vi "Calculate no of Hist bins.vi"(0 "Mean":dbl, 1 "Standard Deviation":dbl, 2 "Time Trace":dbl[](array[numeric]), 3 "Shift Input":T1, 4 "Number of Bins per Sigma":dbl=50.0 format="%#_13g") -> (6 "Shift Output":T1)   [LabVIEW 2022 SP3]
uses:
  Controls/Shift_Cluster.ctl
  Globals/Meas_global.vi
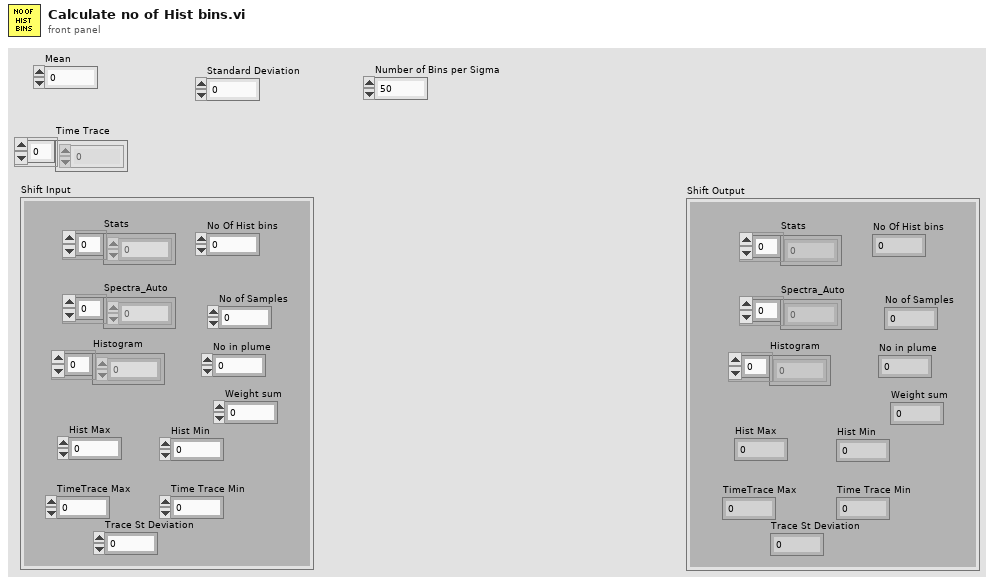
[diagram p1: front panel]
types:
  T1 = typedef "Shift_Cluster.ctl" = cluster{"Stats":dbl[], "Spectra_Auto":dbl[], "Histogram":dbl[], "Hist Max":dbl, "Hist Min":dbl, "No of Samples":i32, "No in plume":i32, "Weight sum":dbl, "No Of Hist bins":i32, "TimeTrace Max":dbl, "Time Trace Min":dbl, "Trace St Deviation":dbl}
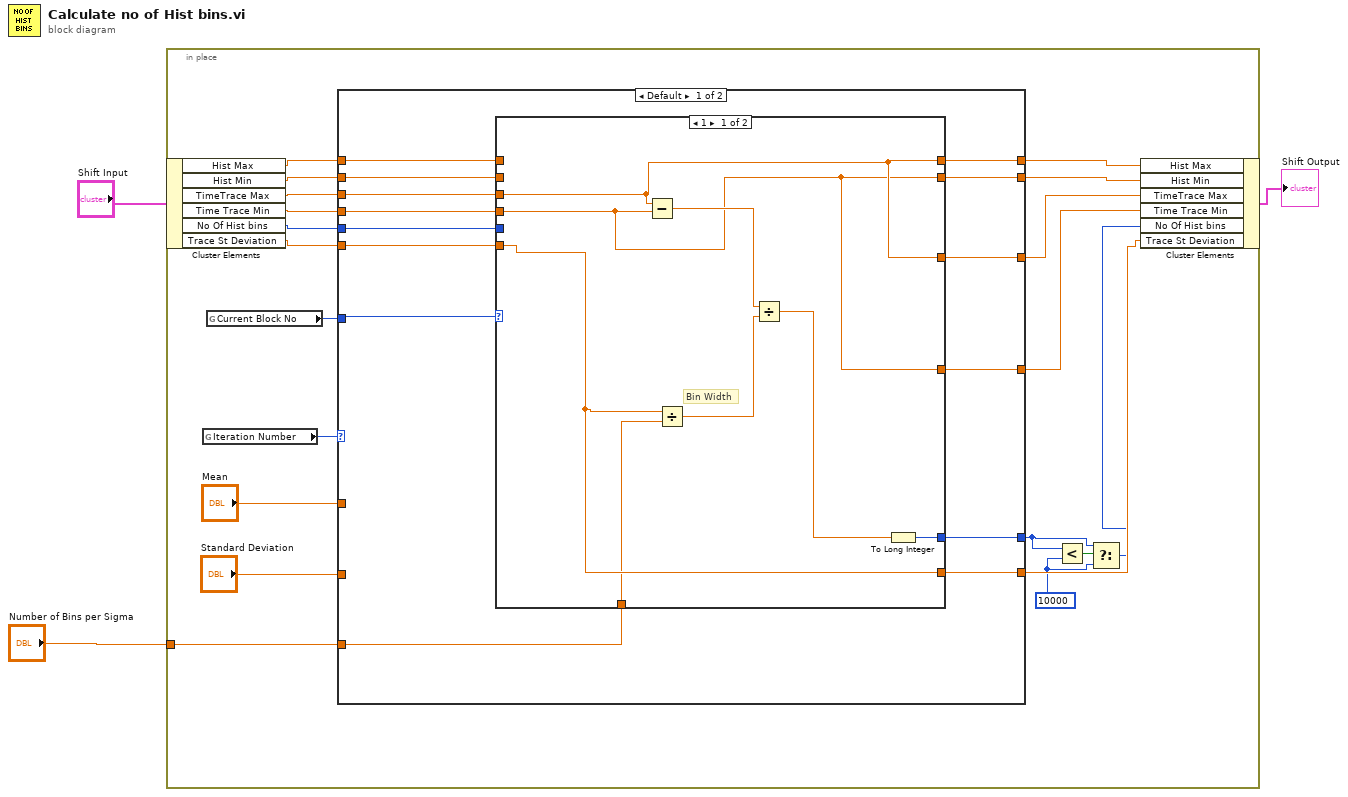
[diagram p0: block diagram]
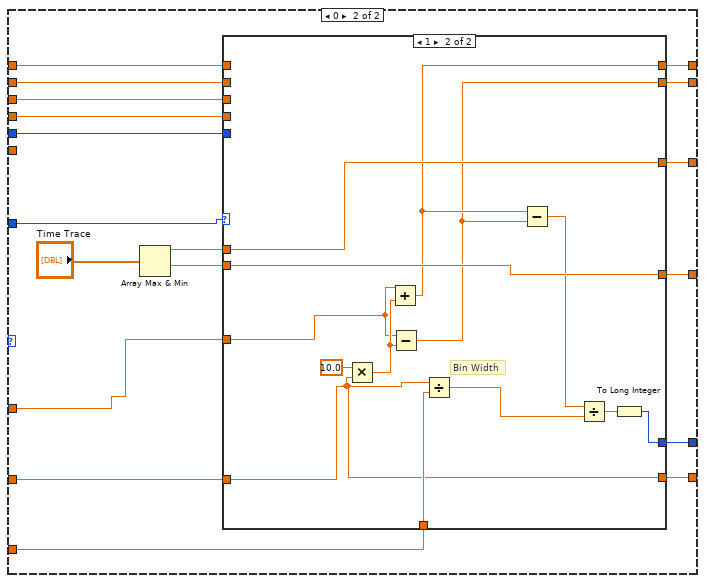
[diagram p3: hidden frame]
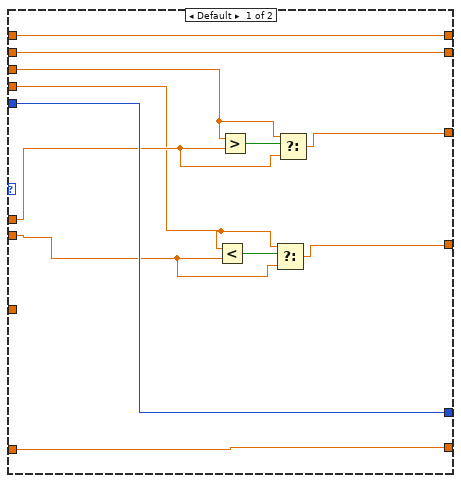
[diagram p4: hidden frame]
diagram:
  n1 = in-place {
    in-place-border: "Number of Bins per Sigma" -> [w10]
    w5 = 10000 ("y")
    n2 = in-place-cluster #1("Shift Input") -> ("Hist Max"=w17:dbl, "Hist Min"=w16:dbl, "TimeTrace Max"=w14:dbl, "Time Trace Min"=w13:dbl, "No Of Hist bins"=w15:i32, "Trace St Deviation"=w11:dbl)
    n3 = global read "Meas_global.vi" "Iteration Number"() -> (w23:i32)
    n4 = global read "Meas_global.vi" "Current Block No"() -> (w22:i32)
    n5 = case shown="Default" w23 {
      tunnel: w22 -> [w37 w68]
      tunnel: [w29 w67] -> w19
      tunnel: [w32 w66] -> w18
      tunnel: [w33 w63] -> w6
      tunnel: [w28 w62] -> w21
      tunnel: [w25 w61] -> w20
      tunnel: w17 -> [w27 w60]
      tunnel: w16 -> [w26 w59]
      tunnel: w15 -> [w34 w58]
      tunnel: w14 -> [w30 w57]
      tunnel: w13 -> [w31 w56]
      tunnel: [w36 w55] -> w12
      tunnel: w11 -> [w35 _]
      tunnel: w10 -> [w24 w54]
      tunnel: "Mean" -> [_ w53]
      tunnel: "Standard Deviation" -> [_ w52]
      frame Default {
        n6 = case shown="1" w37 {
          tunnel: [w41 w51] -> w36
          tunnel: w35 -> [w41 w51]
          tunnel: w34 -> [_ w50]
          tunnel: [w42 w50] -> w33
          tunnel: [w39 w49] -> w32
          tunnel: w31 -> [w39 w49]
          tunnel: w30 -> [w40 w48]
          tunnel: [w40 w48] -> w29
          tunnel: [w40 w47] -> w28
          tunnel: w27 -> [_ w47]
          tunnel: w26 -> [_ w46]
          tunnel: [w39 w46] -> w25
          tunnel: w24 -> [w38 _]
          frame 1 {
            # "Bin Width"
            n7 = Subtract(x=w40, y=w39) -> (x-y=w45:dbl)
            n8 = Divide(x=w41, y=w38) -> (x/y=w44:dbl)
            n9 = Divide(x=w45, y=w44) -> (x/y=w43:dbl)
            n10 = To Long Integer(number=w43) -> (32bit integer=w42:i32)
          }
          frame Default {
          }
        }
      }
      frame 0 {
        n11 = Array Max & Min(array="Time Trace") -> (max value=w65:dbl, min value=w64:dbl)  [unwired: 2 out]
        n12 = case shown="1" w68 {
          tunnel: [w77 w94] -> w67
          tunnel: [w73 w93] -> w66
          tunnel: w65 -> [w75 w94]
          tunnel: w64 -> [w71 w93]
          tunnel: [w79 w89] -> w63
          tunnel: [w81 w86] -> w62
          tunnel: [w80 w85] -> w61
          tunnel: w60 -> [w81 _]
          tunnel: w59 -> [w80 _]
          tunnel: w58 -> [w79 _]
          tunnel: w57 -> [w76 _]
          tunnel: w56 -> [w72 _]
          tunnel: [w70 w82] -> w55
          tunnel: w54 -> [_ w84]
          tunnel: w53 -> [_ w83]
          tunnel: w52 -> [w70 w82]
          frame Default {
            n13 = Less?(x=w72, y=w71) -> (x < y?=w74:bool)
            n14 = Greater?(x=w76, y=w75) -> (0:w78:bool)
            n15 = Select(t=w72, s=w74, f=w71) -> (s? t:f=w73:dbl)
            n16 = Select(t=w76, s=w78, f=w75) -> (s? t:f=w77:dbl)
          }
          frame 1 {
            # "Bin Width"
            n17 = Multiply(x=10.0, y=w82) -> (x*y=w87:dbl)
            n18 = Add(x=w83, y=w87) -> (x+y=w86:dbl)
            n19 = Subtract(x=w83, y=w87) -> (x-y=w85:dbl)
            n20 = Divide(x=w82, y=w84) -> (x/y=w91:dbl)
            n21 = Subtract(x=w86, y=w85) -> (x-y=w92:dbl)
            n22 = Divide(x=w92, y=w91) -> (x/y=w90:dbl)
            n23 = To Long Integer(number=w90) -> (32bit integer=w89:i32)
          }
        }
      }
    }
    n24 = Less?(x=w6, y=w5) -> (x < y?=w7:bool)
    n25 = Select(t=w6, s=w7, f=w5) -> (s? t:f=w4:i32)
    n26 = in-place-cluster #1("Hist Max"=w21, "Hist Min"=w20, "TimeTrace Max"=w19, "Time Trace Min"=w18, "No Of Hist bins"=w4, "Trace St Deviation"=w12) -> (→"Shift Output":T1)
  }
